vi "uTTA_WriteCalibrationFile.vi"(4 "error in":errorcluster, 6 "ucf-File":path, 7 "VISA Refnum in":refnum<visa-resource-name>) -> (0 "error out":errorcluster, 2 "Received":string, 3 "VISA Refnum out":refnum<visa-resource-name>)   [LabVIEW 2021]
uses:
  <vilib>/Utility/config.llb/NI_LVConfig.lvlib
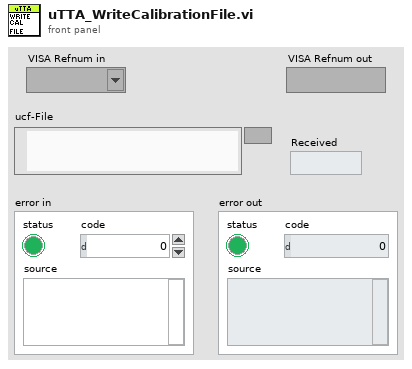
[diagram p1: front panel]
types:
  T1 = typedef "NI_LVConfig.lvlib/Config Data RefNum.ctl" = refnum<k1>
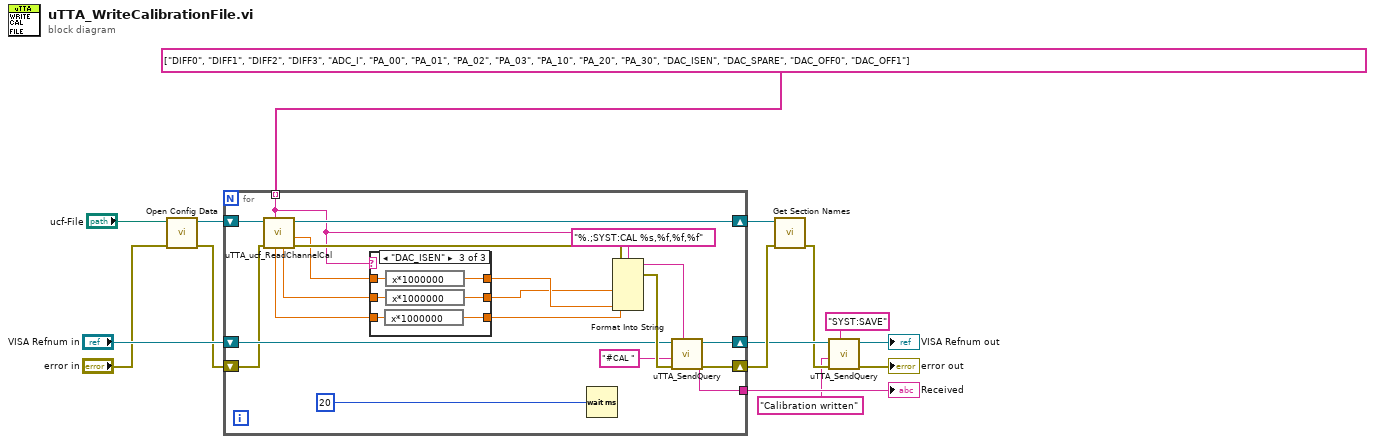
[diagram p0: block diagram]
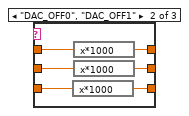
[diagram p3: hidden frame]
diagram:
  n1 = call <vilib>:"Open Config Data.vi"("error in (no error)"="error in", "configuration file path"="ucf-File") -> ("error out"=w8:errorcluster, "refnum"=w13:T1)  [unwired: 7 in, 1 out]
  n2 = for {
    tunnel: [w35] -> w15
    shift-right: [w29] -> w11
    shift-left: w8 -> [w26]
    shift-right: [w30] -> w6
    shift-left: "VISA Refnum in" -> [w31]
    shift-right: [w27] -> w12
    shift-left: w13 -> [w28]
    tunnel: string[] ["DIFF0", "DIFF1", "DIFF2", "DIFF3", "ADC_I", "PA_00", "PA_01", "PA_02", "PA_03", "PA_10", "PA_20", "PA_30", "DAC_ISEN", "DAC_SPARE", "DAC_OFF0", "DAC_OFF1"] -> [w22] mode=indexing
    n3 = call "uTTA_ucf_ReadChannelCal.vi"("Section"=w22, "error in"=w26, "Refnum in"=w28) -> ("error out"=w25:errorcluster, "QuadGain"=w21:dbl, "Refnum out"=w27:T1, "Offset"=w19:dbl, "LinGain"=w17:dbl)  [unwired: 3 in, 1 out]
    n4 = case shown="\"DAC_ISEN\"" w22 {
      tunnel: w21 -> [w38 w42 w48]
      tunnel: w19 -> [w37 w41 w47]
      tunnel: w17 -> [w36 w44 w50]
      tunnel: [w38 w39 w45] -> w20
      tunnel: [w37 w40 w46] -> w18
      tunnel: [w36 w43 w49] -> w16
      frame Default {
      }
      frame "DAC_OFF0", "DAC_OFF1" {
        n5 = expression code="x*1000"(w44) -> (w43:dbl)
        n6 = expression code="x*1000"(w42) -> (w39:dbl)
        n7 = expression code="x*1000"(w41) -> (w40:dbl)
      }
      frame "DAC_ISEN" {
        n8 = expression code="x*1000000"(w50) -> (w49:dbl)
        n9 = expression code="x*1000000"(w48) -> (w45:dbl)
        n10 = expression code="x*1000000"(w47) -> (w46:dbl)
      }
    }
    n11 = Wait (ms)(milliseconds to wait=u32 20) -> ()  [unwired: 1 out]
    n12 = Format Into String(format string="%.;SYST:CAL %s,%f,%f,%f", error in=w25, w22, w18, w16, w20) -> (resulting string=w33:string, error out=w34:errorcluster)  [unwired: 1 in]
    n13 = call "uTTA_SendQuery.vi"("Send String"=w33, "error in (no error)"=w34, "Response Qualifier(\"\")"="#CAL " ("Response Qualifier(\"\")"), "VISA Refnum in"=w31) -> ("error out"=w29:errorcluster, "Received"=w35:string, "VISA Refnum out"=w30:refnum<visa-resource-name>)  [unwired: 5 in]
  }
  "Received" <- w15
  n14 = call <vilib>:"Get Section Names.vi"("error in (no error)"=w11, "refnum"=w12) -> ("error out"=w5:errorcluster)  [unwired: 7 in, 2 out]
  n15 = call "uTTA_SendQuery.vi"("Send String"="SYST:SAVE", "error in (no error)"=w5, "Response Qualifier(\"\")"="Calibration written" ("Response Qualifier(\"\")"), "VISA Refnum in"=w6) -> ("error out"=→"error out":errorcluster, "VISA Refnum out"=→"VISA Refnum out":refnum<visa-resource-name>)  [unwired: 5 in, 1 out]
